vi "FieldOrientedTransform.vi"(7 "Robot Oriented Direction (deg)":dbl, 9 "Joystick Y":dbl, 11 "Joystick X":dbl) -> (1 "Joystick Y'":dbl, 3 "Joystick X'":dbl)   [LabVIEW 2023]
doc: "Transforms X and Y joystick axes based on the robot's current orientation, allowing a swerve robot to be controlled in the field-oriented reference frame. This also allows the driver's frame of reference to be changed arbitrarily to support PoV controls through an arbitrary camera. The code is primarily based on code included in the FRC WPI Library."
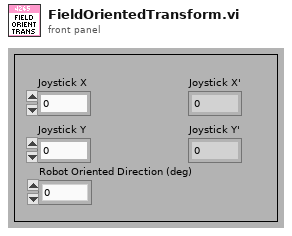
[diagram p1: front panel]
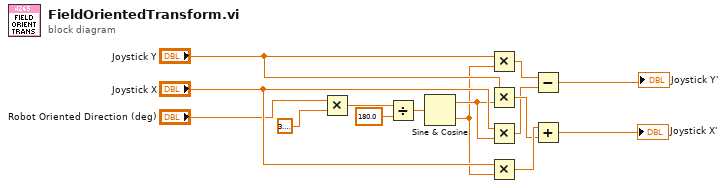
[diagram p0: block diagram]
diagram:
  n1 = Multiply(x="Robot Oriented Direction (deg)", y=3.141592653589793) -> (x*y=w10:dbl)
  n2 = Divide(x=w10, y=180.0) -> (x/y=w9:dbl)
  n3 = Sine & Cosine(0:w9) -> (1:w6:dbl, 2:w5:dbl)
  n4 = Multiply(x="Joystick Y", y=w5) -> (x*y=w4:dbl)
  n5 = Multiply(x="Joystick Y", y=w6) -> (x*y=w7:dbl)
  n6 = Multiply(x="Joystick X", y=w6) -> (x*y=w3:dbl)
  n7 = Multiply(x="Joystick X", y=w5) -> (x*y=w8:dbl)
  n8 = Subtract(x=w4, y=w3) -> (x-y=→"Joystick Y'":dbl)
  n9 = Add(x=w8, y=w7) -> (x+y=→"Joystick X'":dbl)
